vi "Get_PV-1D.vi"(0 "PV Names":string[](array[string]), 1 "variable PV names (F)":bool, 7 "Field Names":string[](array[string]), 9 "Timeout (3)":dbl=3.0, 11 "Error in (no error)":errorcluster, 12 "NoMDEL(F)":bool) -> (4 "PV Names (dup)":string[](array[string]), 6 "1rst Value (string)":string[](array[string]), 8 "1rst Value (number)":dbl[](array[numeric]), 10 "Value Array (number)":dbl[][](array[numeric]), 13 "Status":bool, 14 "PV Info":T1[](array[typedef]), 15 "Error out":errorcluster)   [LabVIEW 2018]
doc: "This is a VI for reading values of EPICS variables.\n\nINPUT:\n <b>PV Name</b>\n name array of EPICS variables\n <b>Field Names</b>\n optional\n string array of EPICS fields (\"EGU\", \"DESCRIPTION\" etc.)\n <b>Timeout (3)</b>\n optional\n timeout for Channel Access requests in seconds\n <b>NoMDEL (F)</b>\n optional\n true: ignore monitor dead-band of Channel Access (EPICS)\n <b>variable PV names (F)</b>\n optional\n true: in case of changing PV names at PV name input (performance drop)\n <b>Error in (no error)</b>\n\nOUTPUT:\n <b>PV Name</b>\n name array of EPICS variables\n <b>1st Value(string)</b>\n value of variable as String\n shows first item of value array\n <b>1st Value(number)</b>\n value of variable as Double\n shows first item of value array\n <b>Value Array(number)</b>\n all values of variable in Double array\n <b>Error out</b>\n <b>PV Info</b>\n cluster array of full answer\n value array(number)\n PV name\n elements\n size of value array\n value array(string)\n all values of variable in string array\n value array(number)\n elements\n size of value array\n status(string)\n status of EPICS PV as String\n status(number)\n status of EPICS PV as Long\n severity(string)\n severity of EPICS PV as String\n severity(number)\n severity of EPICS PV as Long\n time stamp(string)\n stamp of EPICS PV time as String\n time stamp(number)\n stamp of EPICS PV as Long\n field names\n field values\n string array of requsted EPICS field values\n error IO\n <b>Status</b>\n FALSE: request successful\n TRUE: warnings or errors"
uses:
  <userlib>/caLab/PV Info.ctl
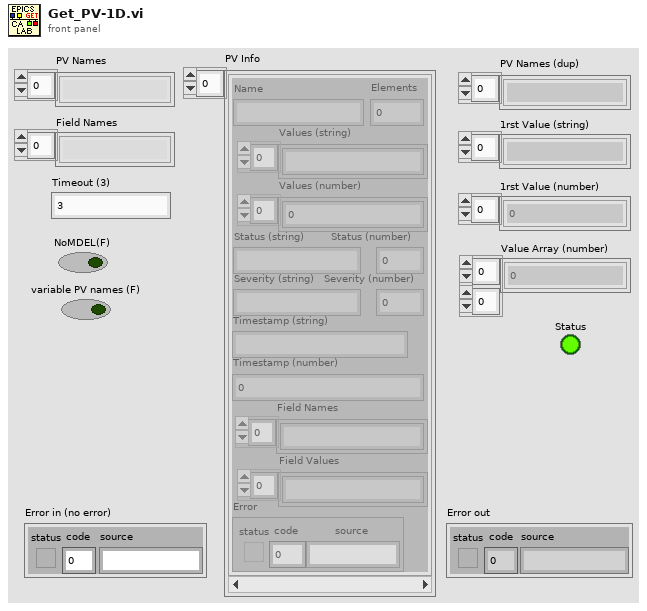
[diagram p1: front panel]
types:
  T1 = typedef "PV Info.ctl" = cluster{"Name":string, "Elements":i32, "Values (string)":string[], "Values (number)":dbl[], "Status (string)":string, "Status (number)":i16, "Severity (string)":string, "Severity (number)":i16, "Timestamp (string)":string, "Timestamp (number)":i32, "Field Names":string[], "Field Values":string[], "Error":errorcluster}
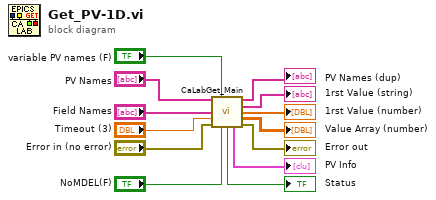
[diagram p0: block diagram]
diagram:
  n1 = call <userlib>:"CaLabGet_Main.vi"("PV Name"="PV Names", "variable PV names (F)"="variable PV names (F)", "Field Names"="Field Names", "Timeout (3)"="Timeout (3)", "error in (no error)"="Error in (no error)", "NoMDEL(F)"="NoMDEL(F)") -> ("PV Name (dup)"=→"PV Names (dup)":string[], "1rst Value (string)"=→"1rst Value (string)":string[], "1rst Value (number)"=→"1rst Value (number)":dbl[], "Value Array (number)"=→"Value Array (number)":dbl[][], "Status"=→"Status":bool, "PV Info"=→"PV Info":T1[], "error out"=→"Error out":errorcluster)  [unwired: 3 out]
